vi "Launch.vi"() -> ()   [LabVIEW 2018]
uses:
  LauncherState.ctl
panel:
  out "Engines":bool
  out "Count":dbl
  in  "Abort":bool
  in  "Launch":bool
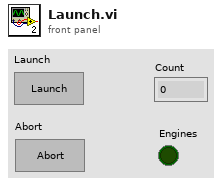
[diagram p1: front panel]
types:
  T1 = typedef "LauncherState.ctl" = enum16{"Ready", "Countdown", "FIre", "Engine Stop", "Abort"}
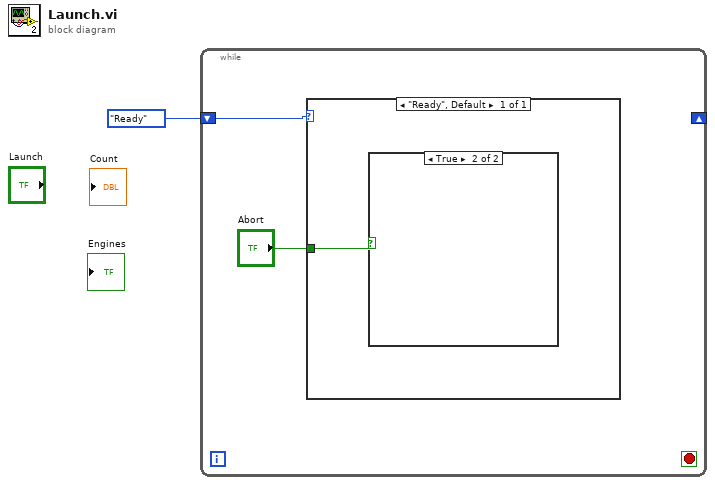
[diagram p0: block diagram]
diagram:
  n1 = while {
    shift-right: _ -> [_]
    shift-left: LauncherState."Ready" ("Launcher State") -> [w3]
    stop <- _ stop-if-true
    n2 = case shown="\"Ready\", Default" w3 {
      tunnel: "Abort" -> [w4]
      frame "Ready", Default {
        n3 = case shown="True" w4 {
          frame False {
          }
          frame True {
          }
        }
      }
    }
  }
